vi "Set Mediator.vi"(8 "error in (no error)":errorcluster caption="错误输入（无错误）", 10 "Mediator":string, 11 "Colleague输入":refnum<class "Colleague.lvclass">) -> (0 "error out":errorcluster caption="错误输出", 3 "Colleague输出":refnum<class "Colleague.lvclass">)   [LabVIEW 2011, in "Colleague.lvclass"]
uses:
  Colleague.lvclass
  Colleague.lvclass/Colleague.ctl
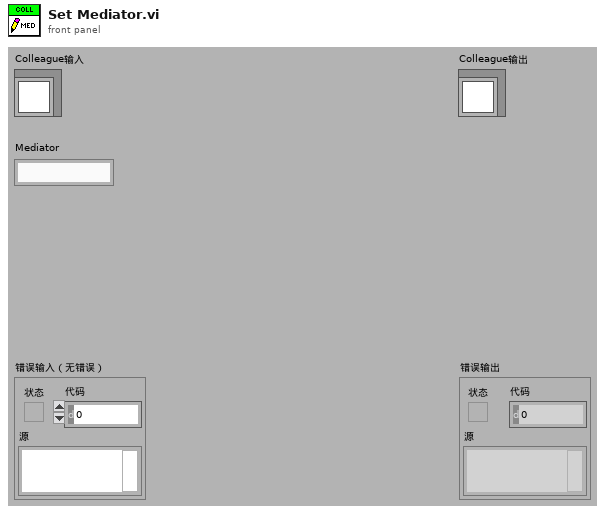
[diagram p1: front panel]
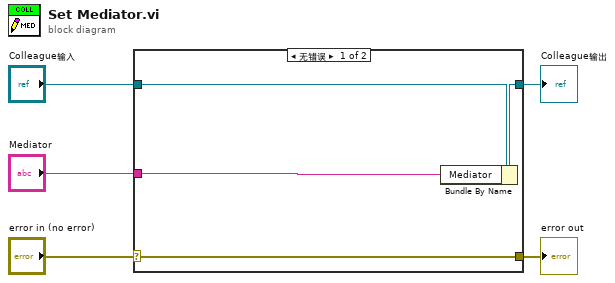
[diagram p0: block diagram]
diagram:
  n1 = case shown="无错误" "error in (no error)" {
    selector: "error in (no error)" -> [w9 w10]
    tunnel: [w9 w10] -> w4
    tunnel: [w7 w11] -> w2
    tunnel: "Colleague输入" -> [w8 w11]
    tunnel: "Mediator" -> [w6 _]
    frame No Error {
      n2 = Bundle By Name(cluster=w8, "Mediator"=w6) -> (w7:refnum<class "Colleague.lvclass">)
    }
    frame Error {
    }
  }
  "error out" <- w4
  "Colleague输出" <- w2
